vi "DE_Three Random Indices.vi"(10 "cur index":i32, 11 "population size":i32) -> (1 "index 2":i32, 2 "index 1":i32, 3 "index 0":i32)   [LabVIEW 2017, in "NI_AAL_GlobalOptimization.lvlib"]
uses:
  <vilib>/gmath/NI_AAL_GlobalOptimization.lvlib
  <vilib>/Analysis/1siggen.llb/Riffle Array (I32) (obs 2012).vi
  <vilib>/Analysis/NI_AALBase.lvlib
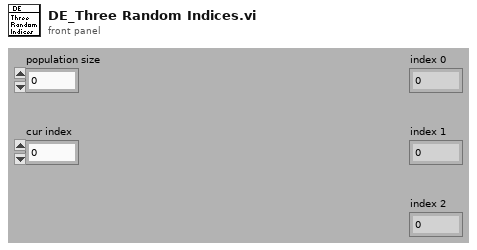
[diagram p1: front panel]
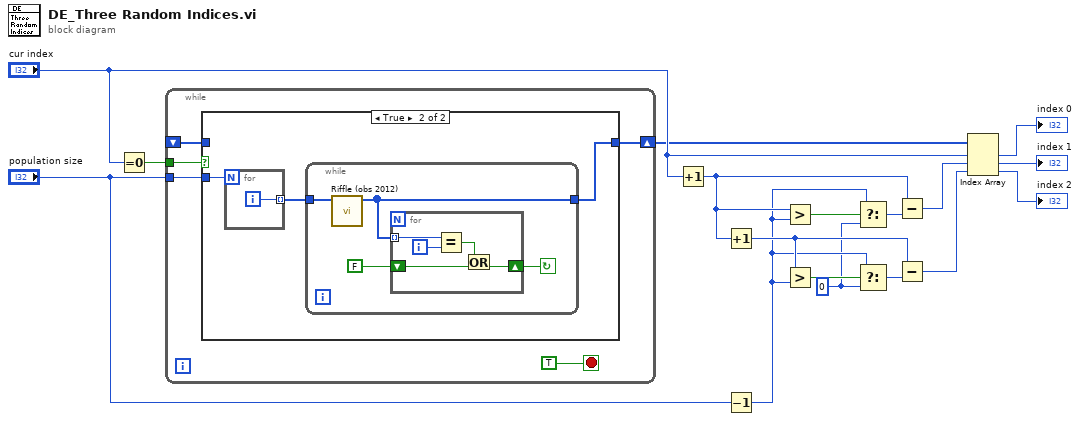
[diagram p0: block diagram]
diagram:
  w1 = 0 ("f")
  n1 = Equal To 0?(x="cur index") -> (x = 0?=w12:bool)
  n2 = while {
    tunnel: w12 -> [w22]
    tunnel: "population size" -> [w21]
    shift-right: [w20] -> w11
    shift-left: _ -> [w19]
    stop <- TRUE stop-if-true
    n3 = case shown="True" w22 {
      tunnel: w21 -> [_ w24]
      tunnel: [w23 w25] -> w20
      tunnel: w19 -> [w23 _]
      frame False {
      }
      frame True {
        n4 = for {
          N: w24 -> [_]
          tunnel: [w36] -> w26 mode=indexing
          i -> [w36]
        }
        n5 = while {
          tunnel: w26 -> [w30]
          tunnel: [w29] -> w25
          stop <- w27 continue-if-true
          n6 = call-poly <vilib>:"Riffle (obs 2012).vi"("X"=w30) -> ("Riffled {X}"=w29:i32[])  [unwired: 8 in, 2 out]
          n7 = for {
            tunnel: w29 -> [w35] mode=indexing
            shift-right: [w31] -> w27
            shift-left: FALSE -> [w32]
            i -> [w34]
            n8 = Equal?(x=w35, y=w34) -> (x = y?=w33:bool)
            n9 = Or(x=w33, y=w32) -> (x .or. y?=w31:bool)
          }
        }
      }
    }
  }
  n10 = Increment(x="cur index") -> (x+1=w8:i32)
  n11 = Increment(x=w8) -> (x+1=w7:i32)
  n12 = Decrement(x="population size") -> (x-1=w2:i32)
  n13 = Greater?(x=w8, y=w2) -> (0:w10:bool)
  n14 = Greater?(x=w7, y=w2) -> (0:w9:bool)
  n15 = Select(t=w2, s=w10, f=w1) -> (s? t:f=w5:i32)
  n16 = Select(t=w2, s=w9, f=w1) -> (s? t:f=w6:i32)
  n17 = Subtract(x=w8, y=w5) -> (x-y=w4:i32)
  n18 = Subtract(x=w7, y=w6) -> (x-y=w3:i32)
  n19 = Index Array(array=w11, index #1="cur index", index #2=w4, index #3=w3) -> (element #1=→"index 0":i32, element #2=→"index 1":i32, element #3=→"index 2":i32)
